vi "Read Lifetime.vi"(11 "Base Actor in":refnum<class "Base Actor.lvclass">) -> (2 "Lifetime":T1=enum."Setup")   [LabVIEW 2020, in "jettl.lvlib" / "Base jettl Actor.lvlib" / "Base Actor.lvlib" / "Base Actor.lvclass"]
uses:
  Base Actor.lvclass
  Lifetime.ctl
  Base Actor.lvclass/Base Actor.ctl
  jettl.lvlib
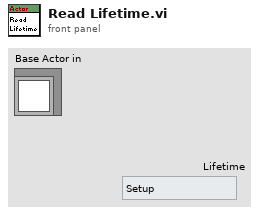
[diagram p1: front panel]
types:
  T1 = typedef "jettl.lvlib/Lifetime.ctl" = enum16{"Init", "Spawn", "Setup", "Teardown Before Started", "Start", "Started", "Stopping With Children", "Stopping Without Children", "Teardown After Started", "Stopped"}
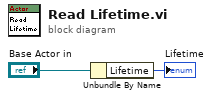
[diagram p0: block diagram]
diagram:
  n1 = Unbundle By Name("Base Actor in") -> ("Lifetime"=→"Lifetime":T1)
